vi "Initialize.vi"(1 "Working":refnum<vi>, 3 "Path to start the search":path) -> (0 "Array":path[](array[path]))   [LabVIEW 2011]
doc: "This VI first checks the path selected. If the path is empty, a File Dialog prompts the user to select a directory. When a path is selected, the VI gets the array of paths of all the files in the selected folder. \nThe VI also sets the \"Working\" LED visible so that the user knows the program has not hung."
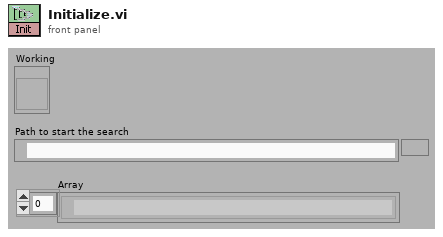
[diagram p1: front panel]
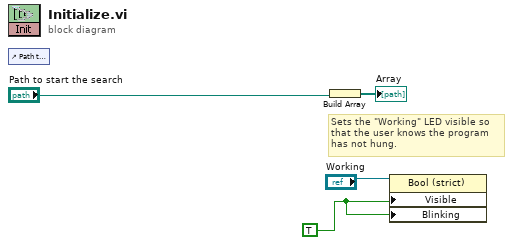
[diagram p0: block diagram]
diagram:
  w2 = TRUE
  # "Sets the \"Working\" LED visible so that the user knows the program has not hung."
  n1 = control-ref of="Path to start the search"() -> ()  [unwired: 1 out]
  n2 = Build Array("Path to start the search") -> (→"Array":path[])
  n3 = property on="Property Node" class="Bool (strict)"(reference="Working", "Visible"=w2, "Blinking"=w2) -> ()  [unwired: 1 in, 2 out]
